vi "create group specification.vi"(8 "error in":errorcluster, 10 "group data dictionary in":refnum<class "data dictionary.lvclass">, 11 "main data dictionary in":refnum<class "data dictionary.lvclass">) -> (0 "error out":errorcluster, 1 "group specification":T1[](array[typedef]), 2 "group data dictionary out":refnum<class "data dictionary.lvclass">, 3 "main data dictionary out":refnum<class "data dictionary.lvclass">)   [LabVIEW 2013, in "tag bus.lvlib" / "data dictionary.lvclass"]
doc: "Uses two data dictionaries and a set of tag names and types to create a group specification. This group specification is a special case of the transfer specification, and can be used to move data from one table to another table. These tables must share the same tags."
uses:
  data dictionary.lvclass
  table/group specification.ctl
  tag/Data Type.ctl
  data dictionary.lvclass/data dictionary.ctl
  lookup polymorphs/locate double.vi
  lookup polymorphs/locate Single.vi
  lookup polymorphs/locate I64.vi
  lookup polymorphs/locate I32.vi
  lookup polymorphs/locate I16.vi
  lookup polymorphs/locate I8.vi
  lookup polymorphs/locate U64.vi
  lookup polymorphs/locate U32.vi
  lookup polymorphs/locate U16.vi
  lookup polymorphs/locate U8.vi
  lookup polymorphs/locate Boolean.vi
  lookup polymorphs/locate String.vi
  lookup polymorphs/locate Array of Double.vi
  lookup polymorphs/locate Array of Single.vi
  lookup polymorphs/locate Array of I64.vi
  lookup polymorphs/locate Array of I32.vi
  lookup polymorphs/locate Array of I16.vi
  lookup polymorphs/locate Array of I8.vi
  lookup polymorphs/locate Array of U64.vi
  lookup polymorphs/locate Array of U32.vi
  lookup polymorphs/locate Array of U16.vi
  lookup polymorphs/locate Array of U8.vi
  lookup polymorphs/locate Array of Boolean.vi
  lookup polymorphs/locate Array of String.vi
  tag/count types.vi
  tag/index to type.vi
  search/find data index.vi
  search/search string list.vi
  tag not found.vi
  tag/tag descriptor.lvclass
  table/data table.lvlib
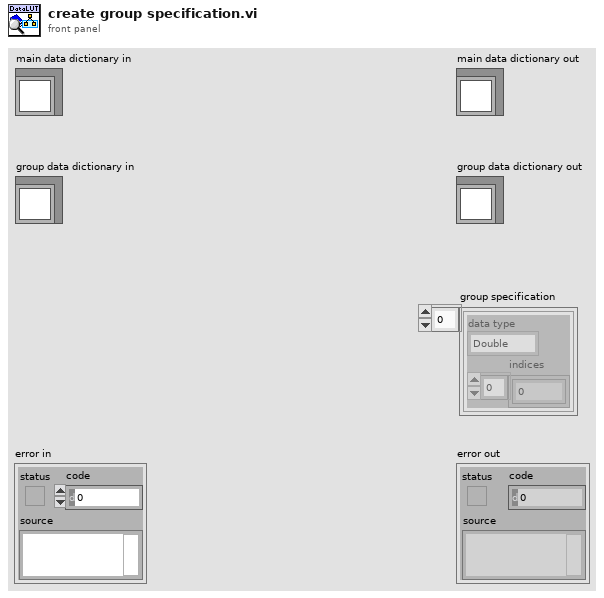
[diagram p1: front panel]
types:
  T1 = typedef "tag bus.lvlib/data table.lvlib/group specification.ctl" = cluster{"data type":T2, "indices":i32[]}
  T2 = typedef "tag bus.lvlib/tag descriptor.lvclass/Data Type.ctl" = enum16{"Double", "Single", "I64", "I32", "I16", "I8", "U64", "U32", "U16", "U8", "Boolean", "String", "Array of Double", "Array of Single", "Array of I64", "Array of I32", "Array of I16", "Array of I8", "Array of U64", "Array of U32", "Array of U16", "Array of U8", "Array of Boolean", "Array of String"}
  T3 = typedef "tag bus.lvlib/binary search.lvlib/sorted list.ctl" = cluster{"sorted strings":string[], "sorted indices":i32[]}
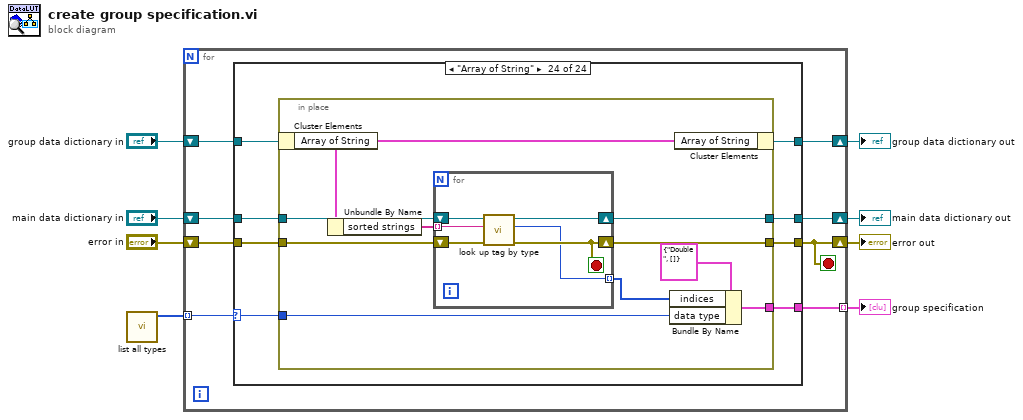
[diagram p0: block diagram]
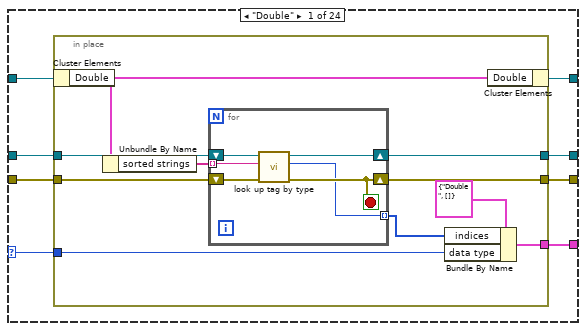
[diagram p2: hidden frame]
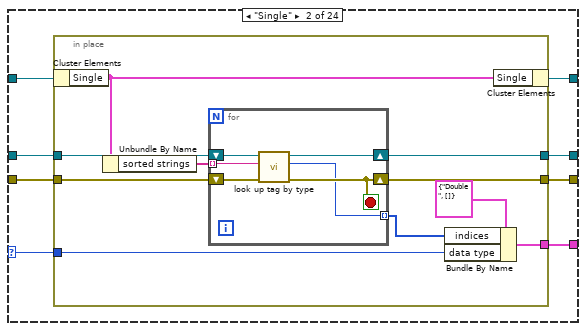
[diagram p3: hidden frame]
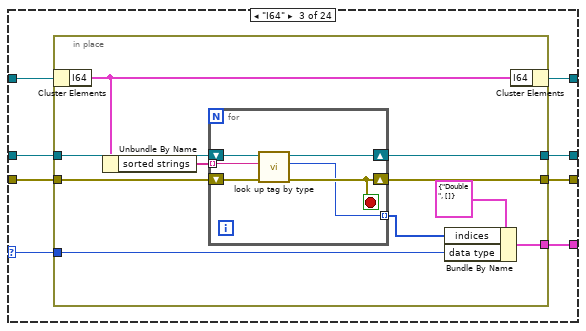
[diagram p4: hidden frame]
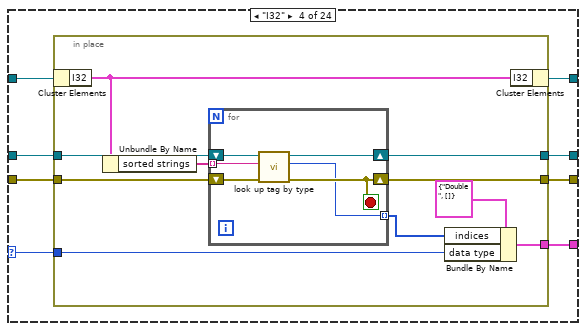
[diagram p5: hidden frame]
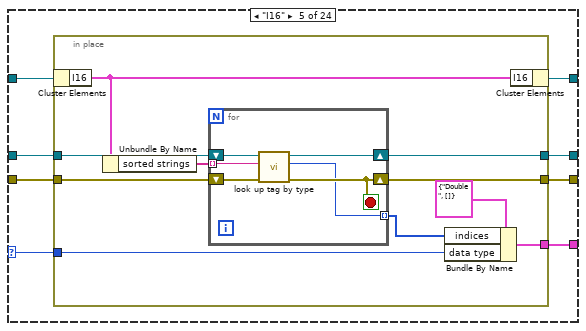
[diagram p6: hidden frame]
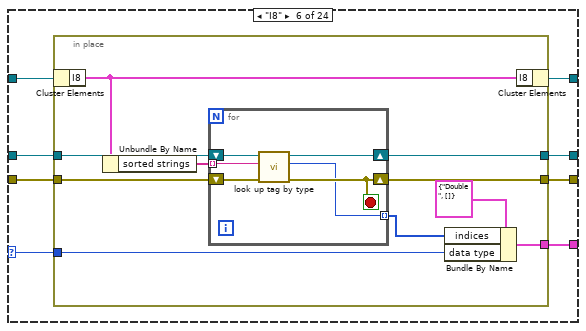
[diagram p7: hidden frame]
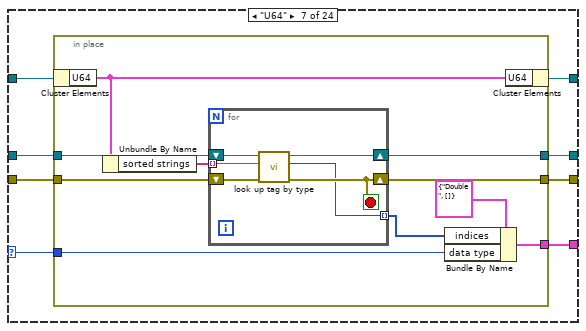
[diagram p8: hidden frame]
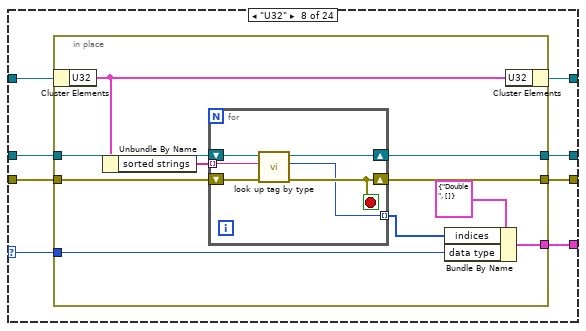
[diagram p9: hidden frame]
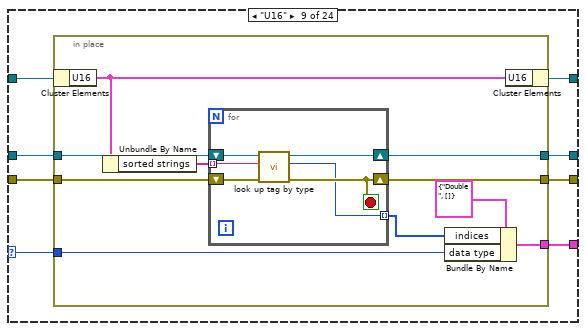
[diagram p10: hidden frame]
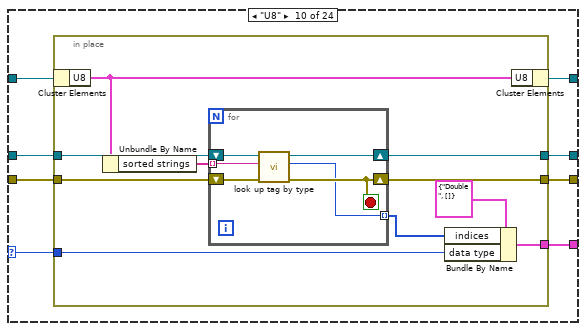
[diagram p11: hidden frame]
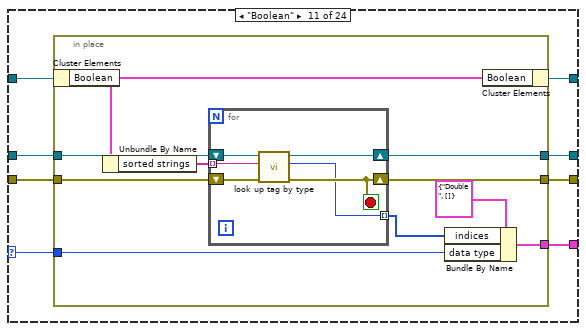
[diagram p12: hidden frame]
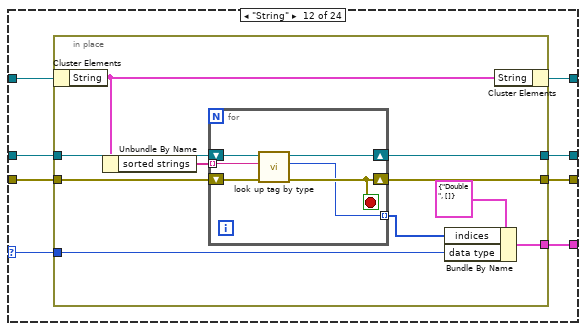
[diagram p13: hidden frame]
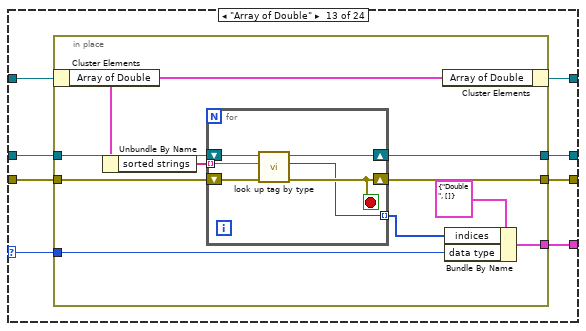
[diagram p14: hidden frame]
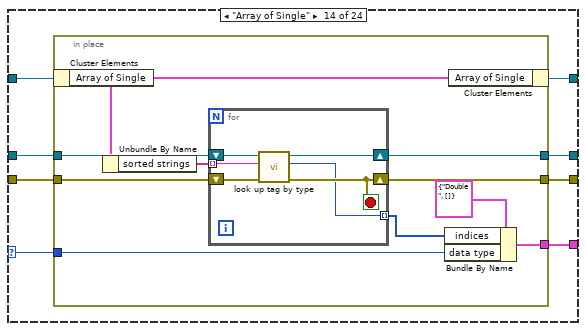
[diagram p15: hidden frame]
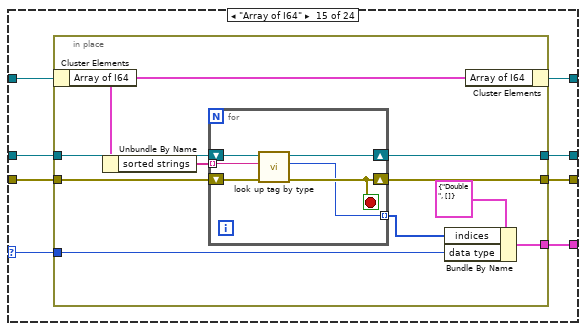
[diagram p16: hidden frame]
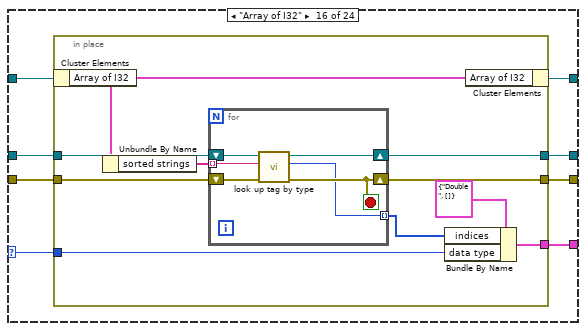
[diagram p17: hidden frame]
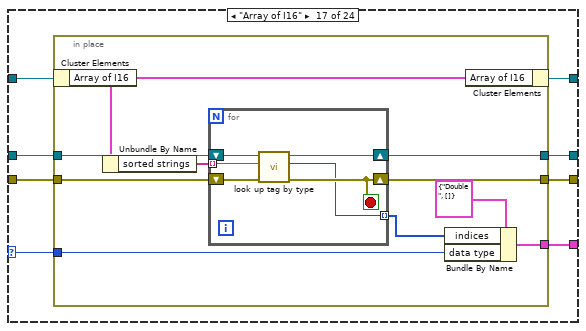
[diagram p18: hidden frame]
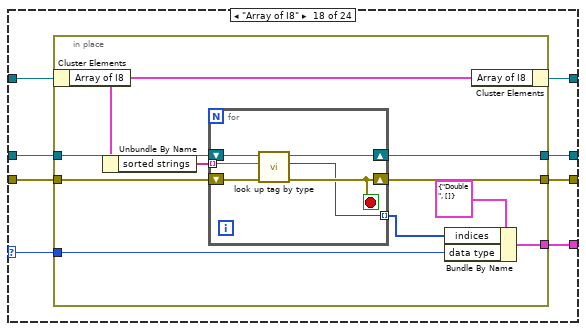
[diagram p19: hidden frame]
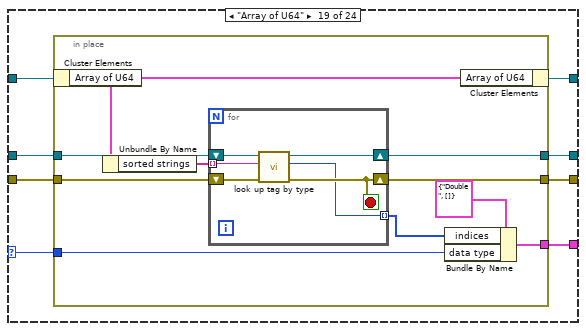
[diagram p20: hidden frame]
diagram:
  n1 = call "list all types.vi"() -> ("all types"=w6:T2[])  [unwired: 11 in]
  n2 = for {
    shift-right: [w11] -> w7
    shift-left: "main data dictionary in" -> [w12]
    tunnel: w6 -> [w16] mode=indexing
    shift-right: [w14] -> w4
    shift-left: "group data dictionary in" -> [w15]
    shift-right: [w9] -> w2
    shift-left: "error in" -> [w13]
    tunnel: [w10] -> w1 mode=indexing
    stop <- w9 stop-if-true
    n3 = case shown="\"Array of String\"" w16 {
      selector: w16 -> [w18 w42 w66 w90 w114 w138 w162 w186 w210 w234 w258 w282 w306 w330 w354 w378 w402 w426 w450 w474 w498 w522 w546 w570]
      tunnel: w15 -> [w24 w48 w72 w96 w120 w144 w168 w192 w216 w240 w264 w288 w312 w336 w360 w384 w408 w432 w456 w480 w504 w528 w552 w576]
      tunnel: [w23 w47 w71 w95 w119 w143 w167 w191 w215 w239 w263 w287 w311 w335 w359 w383 w407 w431 w455 w479 w503 w527 w551 w575] -> w14
      tunnel: w13 -> [w21 w45 w69 w93 w117 w141 w165 w189 w213 w237 w261 w285 w309 w333 w357 w381 w405 w429 w453 w477 w501 w525 w549 w573]
      tunnel: w12 -> [w22 w46 w70 w94 w118 w142 w166 w190 w214 w238 w262 w286 w310 w334 w358 w382 w406 w430 w454 w478 w502 w526 w550 w574]
      tunnel: [w20 w44 w68 w92 w116 w140 w164 w188 w212 w236 w260 w284 w308 w332 w356 w380 w404 w428 w452 w476 w500 w524 w548 w572] -> w11
      tunnel: [w19 w43 w67 w91 w115 w139 w163 w187 w211 w235 w259 w283 w307 w331 w355 w379 w403 w427 w451 w475 w499 w523 w547 w571] -> w9
      tunnel: [w17 w41 w65 w89 w113 w137 w161 w185 w209 w233 w257 w281 w305 w329 w353 w377 w401 w425 w449 w473 w497 w521 w545 w569] -> w10
      frame "Double" {
        n4 = in-place {
          in-place-border: w22 -> [w34]
          in-place-border: w21 -> [w33]
          in-place-border: [w32] -> w20
          in-place-border: [w31] -> w19
          in-place-border: w18 -> [w29]
          in-place-border: [w27] -> w17
          n5 = in-place-cluster #1(w24) -> ("Double"=w26:T3)
          n6 = Unbundle By Name(w26) -> ("sorted strings"=w25:string[])
          n7 = for {
            shift-right: [w37] -> w32
            shift-left: w34 -> [w40]
            tunnel: w25 -> [w38] mode=indexing
            shift-right: [w36] -> w31
            shift-left: w33 -> [w39]
            tunnel: [w35] -> w28 mode=indexing
            stop <- w36 stop-if-true
            n8 = call-poly "look up tag by type.vi"("error in"=w39, "name"=w38, "data dictionary in"=w40) -> ("error out"=w36:errorcluster, "index"=w35:i32, "data dictionary out"=w37:refnum<class "data dictionary.lvclass">)  [unwired: 6 in]
          }
          n9 = Bundle By Name(cluster=T1 {"data type"=enum."Double", "indices"=[]} ("group specification"), "indices"=w28, "data type"=w29) -> (w27:T1)
          n10 = in-place-cluster #1("Double"=w26) -> (w23:refnum<class "data dictionary.lvclass">)
        }
      }
      frame "Single" {
        n11 = in-place {
          in-place-border: w46 -> [w58]
          in-place-border: w45 -> [w57]
          in-place-border: [w56] -> w44
          in-place-border: [w55] -> w43
          in-place-border: w42 -> [w53]
          in-place-border: [w51] -> w41
          n12 = in-place-cluster #2(w48) -> ("Single"=w50:T3)
          n13 = Unbundle By Name(w50) -> ("sorted strings"=w49:string[])
          n14 = for {
            shift-right: [w61] -> w56
            shift-left: w58 -> [w64]
            tunnel: w49 -> [w62] mode=indexing
            shift-right: [w60] -> w55
            shift-left: w57 -> [w63]
            tunnel: [w59] -> w52 mode=indexing
            stop <- w60 stop-if-true
            n15 = call-poly "look up tag by type.vi"("error in"=w63, "name"=w62, "data dictionary in"=w64) -> ("error out"=w60:errorcluster, "index"=w59:i32, "data dictionary out"=w61:refnum<class "data dictionary.lvclass">)  [unwired: 6 in]
          }
          n16 = Bundle By Name(cluster=T1 {"data type"=enum."Double", "indices"=[]} ("group specification"), "indices"=w52, "data type"=w53) -> (w51:T1)
          n17 = in-place-cluster #2("Single"=w50) -> (w47:refnum<class "data dictionary.lvclass">)
        }
      }
      frame "I64" {
        n18 = in-place {
          in-place-border: w70 -> [w82]
          in-place-border: w69 -> [w81]
          in-place-border: [w80] -> w68
          in-place-border: [w79] -> w67
          in-place-border: w66 -> [w77]
          in-place-border: [w75] -> w65
          n19 = in-place-cluster #3(w72) -> ("I64"=w74:T3)
          n20 = Unbundle By Name(w74) -> ("sorted strings"=w73:string[])
          n21 = for {
            shift-right: [w85] -> w80
            shift-left: w82 -> [w88]
            tunnel: w73 -> [w86] mode=indexing
            shift-right: [w84] -> w79
            shift-left: w81 -> [w87]
            tunnel: [w83] -> w76 mode=indexing
            stop <- w84 stop-if-true
            n22 = call-poly "look up tag by type.vi"("error in"=w87, "name"=w86, "data dictionary in"=w88) -> ("error out"=w84:errorcluster, "index"=w83:i32, "data dictionary out"=w85:refnum<class "data dictionary.lvclass">)  [unwired: 6 in]
          }
          n23 = Bundle By Name(cluster=T1 {"data type"=enum."Double", "indices"=[]} ("group specification"), "indices"=w76, "data type"=w77) -> (w75:T1)
          n24 = in-place-cluster #3("I64"=w74) -> (w71:refnum<class "data dictionary.lvclass">)
        }
      }
      frame "I32" {
        n25 = in-place {
          in-place-border: w94 -> [w106]
          in-place-border: w93 -> [w105]
          in-place-border: [w104] -> w92
          in-place-border: [w103] -> w91
          in-place-border: w90 -> [w101]
          in-place-border: [w99] -> w89
          n26 = in-place-cluster #4(w96) -> ("I32"=w98:T3)
          n27 = Unbundle By Name(w98) -> ("sorted strings"=w97:string[])
          n28 = for {
            shift-right: [w109] -> w104
            shift-left: w106 -> [w112]
            tunnel: w97 -> [w110] mode=indexing
            shift-right: [w108] -> w103
            shift-left: w105 -> [w111]
            tunnel: [w107] -> w100 mode=indexing
            stop <- w108 stop-if-true
            n29 = call-poly "look up tag by type.vi"("error in"=w111, "name"=w110, "data dictionary in"=w112) -> ("error out"=w108:errorcluster, "index"=w107:i32, "data dictionary out"=w109:refnum<class "data dictionary.lvclass">)  [unwired: 6 in]
          }
          n30 = Bundle By Name(cluster=T1 {"data type"=enum."Double", "indices"=[]} ("group specification"), "indices"=w100, "data type"=w101) -> (w99:T1)
          n31 = in-place-cluster #4("I32"=w98) -> (w95:refnum<class "data dictionary.lvclass">)
        }
      }
      frame "I16" {
        n32 = in-place {
          in-place-border: w118 -> [w130]
          in-place-border: w117 -> [w129]
          in-place-border: [w128] -> w116
          in-place-border: [w127] -> w115
          in-place-border: w114 -> [w125]
          in-place-border: [w123] -> w113
          n33 = in-place-cluster #5(w120) -> ("I16"=w122:T3)
          n34 = Unbundle By Name(w122) -> ("sorted strings"=w121:string[])
          n35 = for {
            shift-right: [w133] -> w128
            shift-left: w130 -> [w136]
            tunnel: w121 -> [w134] mode=indexing
            shift-right: [w132] -> w127
            shift-left: w129 -> [w135]
            tunnel: [w131] -> w124 mode=indexing
            stop <- w132 stop-if-true
            n36 = call-poly "look up tag by type.vi"("error in"=w135, "name"=w134, "data dictionary in"=w136) -> ("error out"=w132:errorcluster, "index"=w131:i32, "data dictionary out"=w133:refnum<class "data dictionary.lvclass">)  [unwired: 6 in]
          }
          n37 = Bundle By Name(cluster=T1 {"data type"=enum."Double", "indices"=[]} ("group specification"), "indices"=w124, "data type"=w125) -> (w123:T1)
          n38 = in-place-cluster #5("I16"=w122) -> (w119:refnum<class "data dictionary.lvclass">)
        }
      }
      frame "I8" {
        n39 = in-place {
          in-place-border: w142 -> [w154]
          in-place-border: w141 -> [w153]
          in-place-border: [w152] -> w140
          in-place-border: [w151] -> w139
          in-place-border: w138 -> [w149]
          in-place-border: [w147] -> w137
          n40 = in-place-cluster #6(w144) -> ("I8"=w146:T3)
          n41 = Unbundle By Name(w146) -> ("sorted strings"=w145:string[])
          n42 = for {
            shift-right: [w157] -> w152
            shift-left: w154 -> [w160]
            tunnel: w145 -> [w158] mode=indexing
            shift-right: [w156] -> w151
            shift-left: w153 -> [w159]
            tunnel: [w155] -> w148 mode=indexing
            stop <- w156 stop-if-true
            n43 = call-poly "look up tag by type.vi"("error in"=w159, "name"=w158, "data dictionary in"=w160) -> ("error out"=w156:errorcluster, "index"=w155:i32, "data dictionary out"=w157:refnum<class "data dictionary.lvclass">)  [unwired: 6 in]
          }
          n44 = Bundle By Name(cluster=T1 {"data type"=enum."Double", "indices"=[]} ("group specification"), "indices"=w148, "data type"=w149) -> (w147:T1)
          n45 = in-place-cluster #6("I8"=w146) -> (w143:refnum<class "data dictionary.lvclass">)
        }
      }
      frame "U64" {
        n46 = in-place {
          in-place-border: w166 -> [w178]
          in-place-border: w165 -> [w177]
          in-place-border: [w176] -> w164
          in-place-border: [w175] -> w163
          in-place-border: w162 -> [w173]
          in-place-border: [w171] -> w161
          n47 = in-place-cluster #7(w168) -> ("U64"=w170:T3)
          n48 = Unbundle By Name(w170) -> ("sorted strings"=w169:string[])
          n49 = for {
            shift-right: [w181] -> w176
            shift-left: w178 -> [w184]
            tunnel: w169 -> [w182] mode=indexing
            shift-right: [w180] -> w175
            shift-left: w177 -> [w183]
            tunnel: [w179] -> w172 mode=indexing
            stop <- w180 stop-if-true
            n50 = call-poly "look up tag by type.vi"("error in"=w183, "name"=w182, "data dictionary in"=w184) -> ("error out"=w180:errorcluster, "index"=w179:i32, "data dictionary out"=w181:refnum<class "data dictionary.lvclass">)  [unwired: 6 in]
          }
          n51 = Bundle By Name(cluster=T1 {"data type"=enum."Double", "indices"=[]} ("group specification"), "indices"=w172, "data type"=w173) -> (w171:T1)
          n52 = in-place-cluster #7("U64"=w170) -> (w167:refnum<class "data dictionary.lvclass">)
        }
      }
      frame "U32" {
        n53 = in-place {
          in-place-border: w190 -> [w202]
          in-place-border: w189 -> [w201]
          in-place-border: [w200] -> w188
          in-place-border: [w199] -> w187
          in-place-border: w186 -> [w197]
          in-place-border: [w195] -> w185
          n54 = in-place-cluster #8(w192) -> ("U32"=w194:T3)
          n55 = Unbundle By Name(w194) -> ("sorted strings"=w193:string[])
          n56 = for {
            shift-right: [w205] -> w200
            shift-left: w202 -> [w208]
            tunnel: w193 -> [w206] mode=indexing
            shift-right: [w204] -> w199
            shift-left: w201 -> [w207]
            tunnel: [w203] -> w196 mode=indexing
            stop <- w204 stop-if-true
            n57 = call-poly "look up tag by type.vi"("error in"=w207, "name"=w206, "data dictionary in"=w208) -> ("error out"=w204:errorcluster, "index"=w203:i32, "data dictionary out"=w205:refnum<class "data dictionary.lvclass">)  [unwired: 6 in]
          }
          n58 = Bundle By Name(cluster=T1 {"data type"=enum."Double", "indices"=[]} ("group specification"), "indices"=w196, "data type"=w197) -> (w195:T1)
          n59 = in-place-cluster #8("U32"=w194) -> (w191:refnum<class "data dictionary.lvclass">)
        }
      }
      frame "U16" {
        n60 = in-place {
          in-place-border: w214 -> [w226]
          in-place-border: w213 -> [w225]
          in-place-border: [w224] -> w212
          in-place-border: [w223] -> w211
          in-place-border: w210 -> [w221]
          in-place-border: [w219] -> w209
          n61 = in-place-cluster #9(w216) -> ("U16"=w218:T3)
          n62 = Unbundle By Name(w218) -> ("sorted strings"=w217:string[])
          n63 = for {
            shift-right: [w229] -> w224
            shift-left: w226 -> [w232]
            tunnel: w217 -> [w230] mode=indexing
            shift-right: [w228] -> w223
            shift-left: w225 -> [w231]
            tunnel: [w227] -> w220 mode=indexing
            stop <- w228 stop-if-true
            n64 = call-poly "look up tag by type.vi"("error in"=w231, "name"=w230, "data dictionary in"=w232) -> ("error out"=w228:errorcluster, "index"=w227:i32, "data dictionary out"=w229:refnum<class "data dictionary.lvclass">)  [unwired: 6 in]
          }
          n65 = Bundle By Name(cluster=T1 {"data type"=enum."Double", "indices"=[]} ("group specification"), "indices"=w220, "data type"=w221) -> (w219:T1)
          n66 = in-place-cluster #9("U16"=w218) -> (w215:refnum<class "data dictionary.lvclass">)
        }
      }
      frame "U8" {
        n67 = in-place {
          in-place-border: w238 -> [w250]
          in-place-border: w237 -> [w249]
          in-place-border: [w248] -> w236
          in-place-border: [w247] -> w235
          in-place-border: w234 -> [w245]
          in-place-border: [w243] -> w233
          n68 = in-place-cluster #10(w240) -> ("U8"=w242:T3)
          n69 = Unbundle By Name(w242) -> ("sorted strings"=w241:string[])
          n70 = for {
            shift-right: [w253] -> w248
            shift-left: w250 -> [w256]
            tunnel: w241 -> [w254] mode=indexing
            shift-right: [w252] -> w247
            shift-left: w249 -> [w255]
            tunnel: [w251] -> w244 mode=indexing
            stop <- w252 stop-if-true
            n71 = call-poly "look up tag by type.vi"("error in"=w255, "name"=w254, "data dictionary in"=w256) -> ("error out"=w252:errorcluster, "index"=w251:i32, "data dictionary out"=w253:refnum<class "data dictionary.lvclass">)  [unwired: 6 in]
          }
          n72 = Bundle By Name(cluster=T1 {"data type"=enum."Double", "indices"=[]} ("group specification"), "indices"=w244, "data type"=w245) -> (w243:T1)
          n73 = in-place-cluster #10("U8"=w242) -> (w239:refnum<class "data dictionary.lvclass">)
        }
      }
      frame "Boolean" {
        n74 = in-place {
          in-place-border: w262 -> [w274]
          in-place-border: w261 -> [w273]
          in-place-border: [w272] -> w260
          in-place-border: [w271] -> w259
          in-place-border: w258 -> [w269]
          in-place-border: [w267] -> w257
          n75 = in-place-cluster #11(w264) -> ("Boolean"=w266:T3)
          n76 = Unbundle By Name(w266) -> ("sorted strings"=w265:string[])
          n77 = for {
            shift-right: [w277] -> w272
            shift-left: w274 -> [w280]
            tunnel: w265 -> [w278] mode=indexing
            shift-right: [w276] -> w271
            shift-left: w273 -> [w279]
            tunnel: [w275] -> w268 mode=indexing
            stop <- w276 stop-if-true
            n78 = call-poly "look up tag by type.vi"("error in"=w279, "name"=w278, "data dictionary in"=w280) -> ("error out"=w276:errorcluster, "index"=w275:i32, "data dictionary out"=w277:refnum<class "data dictionary.lvclass">)  [unwired: 6 in]
          }
          n79 = Bundle By Name(cluster=T1 {"data type"=enum."Double", "indices"=[]} ("group specification"), "indices"=w268, "data type"=w269) -> (w267:T1)
          n80 = in-place-cluster #11("Boolean"=w266) -> (w263:refnum<class "data dictionary.lvclass">)
        }
      }
      frame "String" {
        n81 = in-place {
          in-place-border: w286 -> [w298]
          in-place-border: w285 -> [w297]
          in-place-border: [w296] -> w284
          in-place-border: [w295] -> w283
          in-place-border: w282 -> [w293]
          in-place-border: [w291] -> w281
          n82 = in-place-cluster #12(w288) -> ("String"=w290:T3)
          n83 = Unbundle By Name(w290) -> ("sorted strings"=w289:string[])
          n84 = for {
            shift-right: [w301] -> w296
            shift-left: w298 -> [w304]
            tunnel: w289 -> [w302] mode=indexing
            shift-right: [w300] -> w295
            shift-left: w297 -> [w303]
            tunnel: [w299] -> w292 mode=indexing
            stop <- w300 stop-if-true
            n85 = call-poly "look up tag by type.vi"("error in"=w303, "name"=w302, "data dictionary in"=w304) -> ("error out"=w300:errorcluster, "index"=w299:i32, "data dictionary out"=w301:refnum<class "data dictionary.lvclass">)  [unwired: 6 in]
          }
          n86 = Bundle By Name(cluster=T1 {"data type"=enum."Double", "indices"=[]} ("group specification"), "indices"=w292, "data type"=w293) -> (w291:T1)
          n87 = in-place-cluster #12("String"=w290) -> (w287:refnum<class "data dictionary.lvclass">)
        }
      }
      frame "Array of Double" {
        n88 = in-place {
          in-place-border: w310 -> [w322]
          in-place-border: w309 -> [w321]
          in-place-border: [w320] -> w308
          in-place-border: [w319] -> w307
          in-place-border: w306 -> [w317]
          in-place-border: [w315] -> w305
          n89 = in-place-cluster #13(w312) -> ("Array of Double"=w314:T3)
          n90 = Unbundle By Name(w314) -> ("sorted strings"=w313:string[])
          n91 = for {
            shift-right: [w325] -> w320
            shift-left: w322 -> [w328]
            tunnel: w313 -> [w326] mode=indexing
            shift-right: [w324] -> w319
            shift-left: w321 -> [w327]
            tunnel: [w323] -> w316 mode=indexing
            stop <- w324 stop-if-true
            n92 = call-poly "look up tag by type.vi"("error in"=w327, "name"=w326, "data dictionary in"=w328) -> ("error out"=w324:errorcluster, "index"=w323:i32, "data dictionary out"=w325:refnum<class "data dictionary.lvclass">)  [unwired: 6 in]
          }
          n93 = in-place-cluster #13("Array of Double"=w314) -> (w311:refnum<class "data dictionary.lvclass">)
          n94 = Bundle By Name(cluster=T1 {"data type"=enum."Double", "indices"=[]} ("group specification"), "indices"=w316, "data type"=w317) -> (w315:T1)
        }
      }
      frame "Array of Single" {
        n95 = in-place {
          in-place-border: w334 -> [w346]
          in-place-border: w333 -> [w345]
          in-place-border: [w344] -> w332
          in-place-border: [w343] -> w331
          in-place-border: w330 -> [w341]
          in-place-border: [w339] -> w329
          n96 = in-place-cluster #14(w336) -> ("Array of Single"=w338:T3)
          n97 = Unbundle By Name(w338) -> ("sorted strings"=w337:string[])
          n98 = for {
            shift-right: [w349] -> w344
            shift-left: w346 -> [w352]
            tunnel: w337 -> [w350] mode=indexing
            shift-right: [w348] -> w343
            shift-left: w345 -> [w351]
            tunnel: [w347] -> w340 mode=indexing
            stop <- w348 stop-if-true
            n99 = call-poly "look up tag by type.vi"("error in"=w351, "name"=w350, "data dictionary in"=w352) -> ("error out"=w348:errorcluster, "index"=w347:i32, "data dictionary out"=w349:refnum<class "data dictionary.lvclass">)  [unwired: 6 in]
          }
          n100 = Bundle By Name(cluster=T1 {"data type"=enum."Double", "indices"=[]} ("group specification"), "indices"=w340, "data type"=w341) -> (w339:T1)
          n101 = in-place-cluster #14("Array of Single"=w338) -> (w335:refnum<class "data dictionary.lvclass">)
        }
      }
      frame "Array of I64" {
        n102 = in-place {
          in-place-border: w358 -> [w370]
          in-place-border: w357 -> [w369]
          in-place-border: [w368] -> w356
          in-place-border: [w367] -> w355
          in-place-border: w354 -> [w365]
          in-place-border: [w363] -> w353
          n103 = in-place-cluster #15(w360) -> ("Array of I64"=w362:T3)
          n104 = Unbundle By Name(w362) -> ("sorted strings"=w361:string[])
          n105 = for {
            shift-right: [w373] -> w368
            shift-left: w370 -> [w376]
            tunnel: w361 -> [w374] mode=indexing
            shift-right: [w372] -> w367
            shift-left: w369 -> [w375]
            tunnel: [w371] -> w364 mode=indexing
            stop <- w372 stop-if-true
            n106 = call-poly "look up tag by type.vi"("error in"=w375, "name"=w374, "data dictionary in"=w376) -> ("error out"=w372:errorcluster, "index"=w371:i32, "data dictionary out"=w373:refnum<class "data dictionary.lvclass">)  [unwired: 6 in]
          }
          n107 = Bundle By Name(cluster=T1 {"data type"=enum."Double", "indices"=[]} ("group specification"), "indices"=w364, "data type"=w365) -> (w363:T1)
          n108 = in-place-cluster #15("Array of I64"=w362) -> (w359:refnum<class "data dictionary.lvclass">)
        }
      }
      frame "Array of I32" {
        n109 = in-place {
          in-place-border: w382 -> [w394]
          in-place-border: w381 -> [w393]
          in-place-border: [w392] -> w380
          in-place-border: [w391] -> w379
          in-place-border: w378 -> [w389]
          in-place-border: [w387] -> w377
          n110 = in-place-cluster #16(w384) -> ("Array of I32"=w386:T3)
          n111 = Unbundle By Name(w386) -> ("sorted strings"=w385:string[])
          n112 = for {
            shift-right: [w397] -> w392
            shift-left: w394 -> [w400]
            tunnel: w385 -> [w398] mode=indexing
            shift-right: [w396] -> w391
            shift-left: w393 -> [w399]
            tunnel: [w395] -> w388 mode=indexing
            stop <- w396 stop-if-true
            n113 = call-poly "look up tag by type.vi"("error in"=w399, "name"=w398, "data dictionary in"=w400) -> ("error out"=w396:errorcluster, "index"=w395:i32, "data dictionary out"=w397:refnum<class "data dictionary.lvclass">)  [unwired: 6 in]
          }
          n114 = Bundle By Name(cluster=T1 {"data type"=enum."Double", "indices"=[]} ("group specification"), "indices"=w388, "data type"=w389) -> (w387:T1)
          n115 = in-place-cluster #16("Array of I32"=w386) -> (w383:refnum<class "data dictionary.lvclass">)
        }
      }
      frame "Array of I16" {
        n116 = in-place {
          in-place-border: w406 -> [w418]
          in-place-border: w405 -> [w417]
          in-place-border: [w416] -> w404
          in-place-border: [w415] -> w403
          in-place-border: w402 -> [w413]
          in-place-border: [w411] -> w401
          n117 = in-place-cluster #17(w408) -> ("Array of I16"=w410:T3)
          n118 = Unbundle By Name(w410) -> ("sorted strings"=w409:string[])
          n119 = for {
            shift-right: [w421] -> w416
            shift-left: w418 -> [w424]
            tunnel: w409 -> [w422] mode=indexing
            shift-right: [w420] -> w415
            shift-left: w417 -> [w423]
            tunnel: [w419] -> w412 mode=indexing
            stop <- w420 stop-if-true
            n120 = call-poly "look up tag by type.vi"("error in"=w423, "name"=w422, "data dictionary in"=w424) -> ("error out"=w420:errorcluster, "index"=w419:i32, "data dictionary out"=w421:refnum<class "data dictionary.lvclass">)  [unwired: 6 in]
          }
          n121 = Bundle By Name(cluster=T1 {"data type"=enum."Double", "indices"=[]} ("group specification"), "indices"=w412, "data type"=w413) -> (w411:T1)
          n122 = in-place-cluster #17("Array of I16"=w410) -> (w407:refnum<class "data dictionary.lvclass">)
        }
      }
      frame "Array of I8" {
        n123 = in-place {
          in-place-border: w430 -> [w442]
          in-place-border: w429 -> [w441]
          in-place-border: [w440] -> w428
          in-place-border: [w439] -> w427
          in-place-border: w426 -> [w437]
          in-place-border: [w435] -> w425
          n124 = in-place-cluster #18(w432) -> ("Array of I8"=w434:T3)
          n125 = Unbundle By Name(w434) -> ("sorted strings"=w433:string[])
          n126 = for {
            shift-right: [w445] -> w440
            shift-left: w442 -> [w448]
            tunnel: w433 -> [w446] mode=indexing
            shift-right: [w444] -> w439
            shift-left: w441 -> [w447]
            tunnel: [w443] -> w436 mode=indexing
            stop <- w444 stop-if-true
            n127 = call-poly "look up tag by type.vi"("error in"=w447, "name"=w446, "data dictionary in"=w448) -> ("error out"=w444:errorcluster, "index"=w443:i32, "data dictionary out"=w445:refnum<class "data dictionary.lvclass">)  [unwired: 6 in]
          }
          n128 = Bundle By Name(cluster=T1 {"data type"=enum."Double", "indices"=[]} ("group specification"), "indices"=w436, "data type"=w437) -> (w435:T1)
          n129 = in-place-cluster #18("Array of I8"=w434) -> (w431:refnum<class "data dictionary.lvclass">)
        }
      }
      frame "Array of U64" {
        n130 = in-place {
          in-place-border: w454 -> [w466]
          in-place-border: w453 -> [w465]
          in-place-border: [w464] -> w452
          in-place-border: [w463] -> w451
          in-place-border: w450 -> [w461]
          in-place-border: [w459] -> w449
          n131 = in-place-cluster #19(w456) -> ("Array of U64"=w458:T3)
          n132 = Unbundle By Name(w458) -> ("sorted strings"=w457:string[])
          n133 = for {
            shift-right: [w469] -> w464
            shift-left: w466 -> [w472]
            tunnel: w457 -> [w470] mode=indexing
            shift-right: [w468] -> w463
            shift-left: w465 -> [w471]
            tunnel: [w467] -> w460 mode=indexing
            stop <- w468 stop-if-true
            n134 = call-poly "look up tag by type.vi"("error in"=w471, "name"=w470, "data dictionary in"=w472) -> ("error out"=w468:errorcluster, "index"=w467:i32, "data dictionary out"=w469:refnum<class "data dictionary.lvclass">)  [unwired: 6 in]
          }
          n135 = Bundle By Name(cluster=T1 {"data type"=enum."Double", "indices"=[]} ("group specification"), "indices"=w460, "data type"=w461) -> (w459:T1)
          n136 = in-place-cluster #19("Array of U64"=w458) -> (w455:refnum<class "data dictionary.lvclass">)
        }
      }
      frame "Array of U32" {
        n137 = in-place {
          in-place-border: w478 -> [w490]
          in-place-border: w477 -> [w489]
          in-place-border: [w488] -> w476
          in-place-border: [w487] -> w475
          in-place-border: w474 -> [w485]
          in-place-border: [w483] -> w473
          n138 = in-place-cluster #20(w480) -> ("Array of U32"=w482:T3)
          n139 = Unbundle By Name(w482) -> ("sorted strings"=w481:string[])
          n140 = for {
            shift-right: [w493] -> w488
            shift-left: w490 -> [w496]
            tunnel: w481 -> [w494] mode=indexing
            shift-right: [w492] -> w487
            shift-left: w489 -> [w495]
            tunnel: [w491] -> w484 mode=indexing
            stop <- w492 stop-if-true
            n141 = call-poly "look up tag by type.vi"("error in"=w495, "name"=w494, "data dictionary in"=w496) -> ("error out"=w492:errorcluster, "index"=w491:i32, "data dictionary out"=w493:refnum<class "data dictionary.lvclass">)  [unwired: 6 in]
          }
          n142 = Bundle By Name(cluster=T1 {"data type"=enum."Double", "indices"=[]} ("group specification"), "indices"=w484, "data type"=w485) -> (w483:T1)
          n143 = in-place-cluster #20("Array of U32"=w482) -> (w479:refnum<class "data dictionary.lvclass">)
        }
      }
      frame "Array of U16" {
        n144 = in-place {
          in-place-border: w502 -> [w514]
          in-place-border: w501 -> [w513]
          in-place-border: [w512] -> w500
          in-place-border: [w511] -> w499
          in-place-border: w498 -> [w509]
          in-place-border: [w507] -> w497
          n145 = in-place-cluster #21(w504) -> ("Array of U16"=w506:T3)
          n146 = Unbundle By Name(w506) -> ("sorted strings"=w505:string[])
          n147 = for {
            shift-right: [w517] -> w512
            shift-left: w514 -> [w520]
            tunnel: w505 -> [w518] mode=indexing
            shift-right: [w516] -> w511
            shift-left: w513 -> [w519]
            tunnel: [w515] -> w508 mode=indexing
            stop <- w516 stop-if-true
            n148 = call-poly "look up tag by type.vi"("error in"=w519, "name"=w518, "data dictionary in"=w520) -> ("error out"=w516:errorcluster, "index"=w515:i32, "data dictionary out"=w517:refnum<class "data dictionary.lvclass">)  [unwired: 6 in]
          }
          n149 = Bundle By Name(cluster=T1 {"data type"=enum."Double", "indices"=[]} ("group specification"), "indices"=w508, "data type"=w509) -> (w507:T1)
          n150 = in-place-cluster #21("Array of U16"=w506) -> (w503:refnum<class "data dictionary.lvclass">)
        }
      }
      frame "Array of U8" {
        n151 = in-place {
          in-place-border: w526 -> [w538]
          in-place-border: w525 -> [w537]
          in-place-border: [w536] -> w524
          in-place-border: [w535] -> w523
          in-place-border: w522 -> [w533]
          in-place-border: [w531] -> w521
          n152 = in-place-cluster #22(w528) -> ("Array of U8"=w530:T3)
          n153 = Unbundle By Name(w530) -> ("sorted strings"=w529:string[])
          n154 = for {
            shift-right: [w541] -> w536
            shift-left: w538 -> [w544]
            tunnel: w529 -> [w542] mode=indexing
            shift-right: [w540] -> w535
            shift-left: w537 -> [w543]
            tunnel: [w539] -> w532 mode=indexing
            stop <- w540 stop-if-true
            n155 = call-poly "look up tag by type.vi"("error in"=w543, "name"=w542, "data dictionary in"=w544) -> ("error out"=w540:errorcluster, "index"=w539:i32, "data dictionary out"=w541:refnum<class "data dictionary.lvclass">)  [unwired: 6 in]
          }
          n156 = Bundle By Name(cluster=T1 {"data type"=enum."Double", "indices"=[]} ("group specification"), "indices"=w532, "data type"=w533) -> (w531:T1)
          n157 = in-place-cluster #22("Array of U8"=w530) -> (w527:refnum<class "data dictionary.lvclass">)
        }
      }
      frame "Array of Boolean" {
        n158 = in-place {
          in-place-border: w550 -> [w562]
          in-place-border: w549 -> [w561]
          in-place-border: [w560] -> w548
          in-place-border: [w559] -> w547
          in-place-border: w546 -> [w557]
          in-place-border: [w555] -> w545
          n159 = in-place-cluster #23(w552) -> ("Array of Boolean"=w554:T3)
          n160 = Unbundle By Name(w554) -> ("sorted strings"=w553:string[])
          n161 = for {
            shift-right: [w565] -> w560
            shift-left: w562 -> [w568]
            tunnel: w553 -> [w566] mode=indexing
            shift-right: [w564] -> w559
            shift-left: w561 -> [w567]
            tunnel: [w563] -> w556 mode=indexing
            stop <- w564 stop-if-true
            n162 = call-poly "look up tag by type.vi"("error in"=w567, "name"=w566, "data dictionary in"=w568) -> ("error out"=w564:errorcluster, "index"=w563:i32, "data dictionary out"=w565:refnum<class "data dictionary.lvclass">)  [unwired: 6 in]
          }
          n163 = in-place-cluster #23("Array of Boolean"=w554) -> (w551:refnum<class "data dictionary.lvclass">)
          n164 = Bundle By Name(cluster=T1 {"data type"=enum."Double", "indices"=[]} ("group specification"), "indices"=w556, "data type"=w557) -> (w555:T1)
        }
      }
      frame "Array of String" {
        n165 = in-place {
          in-place-border: w574 -> [w586]
          in-place-border: w573 -> [w585]
          in-place-border: [w584] -> w572
          in-place-border: [w583] -> w571
          in-place-border: w570 -> [w581]
          in-place-border: [w579] -> w569
          n166 = in-place-cluster #24(w576) -> ("Array of String"=w578:T3)
          n167 = Unbundle By Name(w578) -> ("sorted strings"=w577:string[])
          n168 = for {
            shift-right: [w589] -> w584
            shift-left: w586 -> [w592]
            tunnel: w577 -> [w590] mode=indexing
            shift-right: [w588] -> w583
            shift-left: w585 -> [w591]
            tunnel: [w587] -> w580 mode=indexing
            stop <- w588 stop-if-true
            n169 = call-poly "look up tag by type.vi"("error in"=w591, "name"=w590, "data dictionary in"=w592) -> ("error out"=w588:errorcluster, "index"=w587:i32, "data dictionary out"=w589:refnum<class "data dictionary.lvclass">)  [unwired: 6 in]
          }
          n170 = Bundle By Name(cluster=T1 {"data type"=enum."Double", "indices"=[]} ("group specification"), "indices"=w580, "data type"=w581) -> (w579:T1)
          n171 = in-place-cluster #24("Array of String"=w578) -> (w575:refnum<class "data dictionary.lvclass">)
        }
      }
    }
  }
  "error out" <- w2
  "main data dictionary out" <- w7
  "group data dictionary out" <- w4
  "group specification" <- w1
